vi "获取当前PCB拍照点位信息.vi"(10 "当前第几片PCB":i32) -> (0 "自动锁螺丝: 锁螺丝相对拍照时旋转角度-单片PCB":i32[](array[numeric]), 1 "单片PCB补偿量":T1[](array[typedef]), 2 "当前PCB实际拍照点":T2[](array[typedef]), 4 "放料点相对拍照点高度差(数组)":dbl[](array[numeric]))   [LabVIEW 2014]
uses:
  Controls/XYZRPos.ctl
  Controls/XYZPos.ctl
  Global.vi
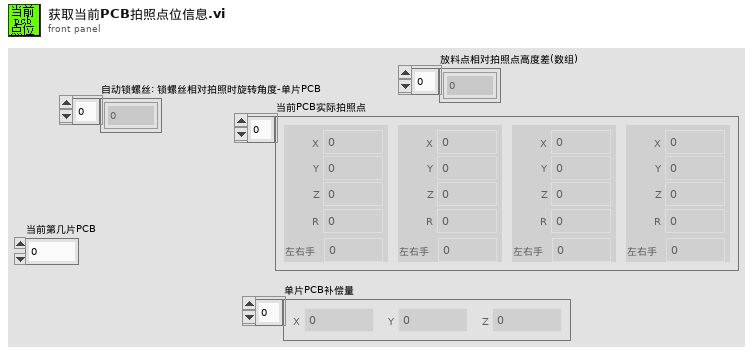
[diagram p1: front panel]
types:
  T1 = typedef "XYZPos.ctl" = cluster{"X":dbl, "Y":dbl, "Z":dbl}
  T2 = typedef "XYZRPos+左右手.ctl" = cluster{"坐标":T3, "左右手":dbl}
  T3 = typedef "XYZRPos.ctl" = cluster{"X":dbl, "Y":dbl, "Z":dbl, "R":dbl}
  T4 = typedef "ModeEditeControl.ctl" = cluster{"Root":path, "AllModelFold":path, "AllModelNamePath":path, "所有零件型号":string[], "当前零件型号":string, "所有建立零件信息":string[][], "当前零件序号":i32, "当前产品所有点位信息":cluster{"当前点位序号":i32, "点位信息路径":path, "CAD点位坐标路径":path, "点位信息表":string[][], "当前点位信息":T5, "CAD图纸点位个数":i32}, "当前产品信息":T7, "所有螺丝和垫片型号Path":path, "Mark拍照点坐标":T2[][], "自动锁螺丝: PCB孔拍照点-多片PCB(去除未勾选的)":T2[], "8个供料盘是否供料-1PCB(去除未勾选的)":bool[], "8个供料盘是否拍照取料":bool[], "自动锁螺丝: 1PCB每颗螺丝来自哪个供料盘U8(去除未勾选的)":u8[], "自动锁螺丝: 1PCB每颗螺丝拧紧程式编号U8(去除未勾选的)":u8[], "4个预锁程式+4个复锁程式编号U8":u8[], "自动锁螺丝: 锁螺丝相对拍照时旋转角度-多片PCB(去除未勾选的)":i32[], "自动锁螺丝: 点位补偿值-多片PCB(去除未勾选的)":T1[], "1PCB上自动锁螺丝个数(去除未勾选的)":i32, "自动锁螺丝: 放料点相对拍照点高度差-多片PCB(去除未勾选的)":dbl[], "8个供料盘是否供料(包括未勾选的)":bool[], "已勾选的自动锁螺丝点位供料盘设定错误":bool, "自动锁螺丝: 复锁拍照点-多片PCB(去除未勾选的)":T2[][], "自动锁螺丝: 1PCB每颗螺丝外径*10(去除未勾选的)":u32[], "拧紧程式参数":cluster{"所有拧紧程式参数表路径":path, "所有拧紧程式参数表":string[][], "自动锁螺丝: 每个托盘螺丝拧紧程式参数":T10[], "自动锁螺丝: 预锁复锁拧紧程式参数":T10[], "所有拧紧程式参数表当前行":i32}, "已勾选的自动锁螺丝点位拧紧程式序号设定错误":bool}
  T5 = typedef "锁附点位信息.ctl" = cluster{"点位名称":string, "点位坐标(图纸)":T1, "点位坐标(实际)":T3, "补偿值":T1, "锁附时机械手角度":T6, "放料点相对Mark\n拍照点高度差":dbl, "选择螺丝托盘":enum32{"托盘1", "托盘2", "托盘3", "托盘4", "托盘5", "托盘6", "托盘7", "托盘8"}, "拧紧程式序号":u16, "预锁程式序号":u16, "复锁程式序号":u16, "自动锁螺丝":bool}
  T6 = typedef "锁附时机械手角度.ctl" = enum16{"0度", "顺时针90度", "顺时针180度", "逆时针90度", "逆时针180度"}
  T7 = typedef "ModelInfo.ctl" = cluster{"产品型号":string, "螺丝刀型号":T8, "载具上放几片PCB":u16, "1片PCB锁几颗螺丝":u16, "CAD点位坐标文档路径":path, "托盘1螺丝型号":T9, "托盘2螺丝型号":T9, "托盘3螺丝型号":T9, "托盘4螺丝型号":T9, "托盘5螺丝型号":T9, "托盘6螺丝型号":T9, "托盘7螺丝型号":T9, "托盘8螺丝型号":T9, "托盘1螺丝锁紧程式序号":u32, "托盘2螺丝锁紧程式序号":u32, "托盘3螺丝锁紧程式序号":u32, "托盘4螺丝锁紧程式序号":u32, "托盘5螺丝锁紧程式序号":u32, "托盘6螺丝锁紧程式序号":u32, "托盘7螺丝锁紧程式序号":u32, "托盘8螺丝锁紧程式序号":u32, "预锁程式序号":u32, "复锁程式序号":u32, "复锁拍照点与Mark拍照点高度差":dbl, "取料点与P2高度差":dbl, "拍PCB孔曝光时间":u32, "取料拍螺帽曝光时间":u32, "复锁拍螺帽曝光时间":u32, "下相机曝光时间":u32}
  T8 = typedef "螺丝刀类型.ctl" = enum16{"螺丝刀1-1*3mm", "螺丝刀2-1.5*3mm", "螺丝刀3-2*3mm", "螺丝刀4-2*4mm", "螺丝刀5-2.5*4mm"}
  T9 = typedef "控件-螺丝型号.ctl" = enum16{"不供料", "一字螺丝M2.5*4", "一字螺丝M2.5*6", "一字螺丝M2.5*8", "一字螺丝M2.5*10", "一字螺丝M2.5*12", "一字螺丝M2.5*14", "一字螺丝M2.5*16", "一字螺丝M2.5*18", "一字螺丝M2.5*20", "一字螺丝M3*4", "一字螺丝M3*6", "一字螺丝M3*8", "一字螺丝M3*10", "一字螺丝M3*12", "一字螺丝M3*14", "一字螺丝M3*16", "一字螺丝M3*18", "一字螺丝M3*20", "一字螺丝M4*6", "一字螺丝M4*8", "一字螺丝M4*10", "一字螺丝M4*12", "一字螺丝M4*14", "一字螺丝M4*16", "一字螺丝M4*18", "一字螺丝M4*20", "十字螺丝M2.5*4", "十字螺丝M2.5*6", "十字螺丝M2.5*8", "十字螺丝M2.5*10", "十字螺丝M2.5*12", "十字螺丝M2.5*14", "十字螺丝M2.5*16", "十字螺丝M2.5*18", "十字螺丝M2.5*20", "十字螺丝M3*4", "十字螺丝M3*6", "十字螺丝M3*8", "十字螺丝M3*10", "十字螺丝M3*12", "十字螺丝M3*14", "十字螺丝M3*16", "十字螺丝M3*18", "十字螺丝M3*20", "十字螺丝M4*6", "十字螺丝M4*8", "十字螺丝M4*10", "十字螺丝M4*12", "十字螺丝M4*14", "十字螺丝M4*16", "十字螺丝M4*18", "十字螺丝M4*20"}
  T10 = typedef "控件-拧紧程式参数.ctl" = cluster{"螺距":dbl, "入牙段转速":dbl, "入牙段转角":dbl, "快速段转速":dbl, "快速段转角":dbl, "快速段Z补偿":dbl, "拧紧转速":dbl}
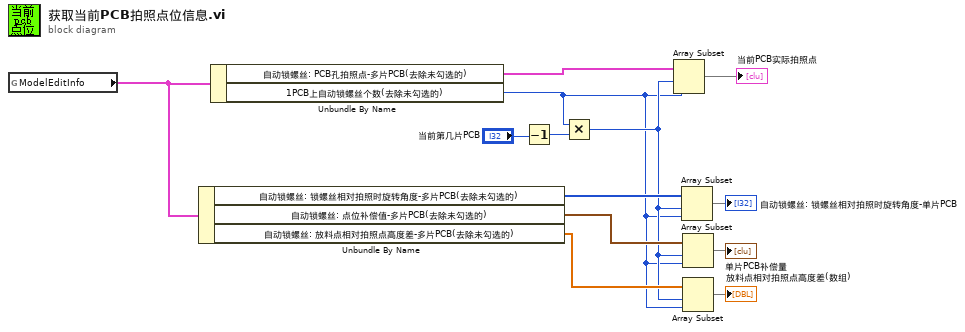
[diagram p0: block diagram]
diagram:
  n1 = global read "Global.vi" "ModelEditInfo"() -> (w10:T4)
  n2 = Unbundle By Name(w10) -> ("自动锁螺丝: 锁螺丝相对拍照时旋转角度-多片PCB(去除未勾选的)"=w8:i32[], "自动锁螺丝: 点位补偿值-多片PCB(去除未勾选的)"=w6:T1[], "自动锁螺丝: 放料点相对拍照点高度差-多片PCB(去除未勾选的)"=w4:dbl[])
  n3 = Unbundle By Name(w10) -> ("自动锁螺丝: PCB孔拍照点-多片PCB(去除未勾选的)"=w11:T2[], "1PCB上自动锁螺丝个数(去除未勾选的)"=w2:i32)
  n4 = Decrement(x="当前第几片PCB") -> (x-1=w13:i32)
  n5 = Multiply(x=w2, y=w13) -> (x*y=w3:i32)
  n6 = Array Subset(array=w11, index=w3, length=w2) -> (→"当前PCB实际拍照点":T2[])
  n7 = Array Subset(array=w8, index=w3, length=w2) -> (→"自动锁螺丝: 锁螺丝相对拍照时旋转角度-单片PCB":i32[])
  n8 = Array Subset(array=w6, index=w3, length=w2) -> (→"单片PCB补偿量":T1[])
  n9 = Array Subset(array=w4, index=w3, length=w2) -> (→"放料点相对拍照点高度差(数组)":dbl[])
